vi "数据地址解析.vi"(7 "输入数据":string, 8 "错误输入（无错误）":errorcluster, 9 "地址判断位":bool, 10 "上轮成功输入时间":timestamp, 11 "回传数据队列":refnum<queue>) -> (0 "错误输出":errorcluster, 1 "输出时间":timestamp, 2 "数据状态":string, 3 "回传数据队列":refnum<queue>, 5 "超时标志位":bool)   [LabVIEW 2020]
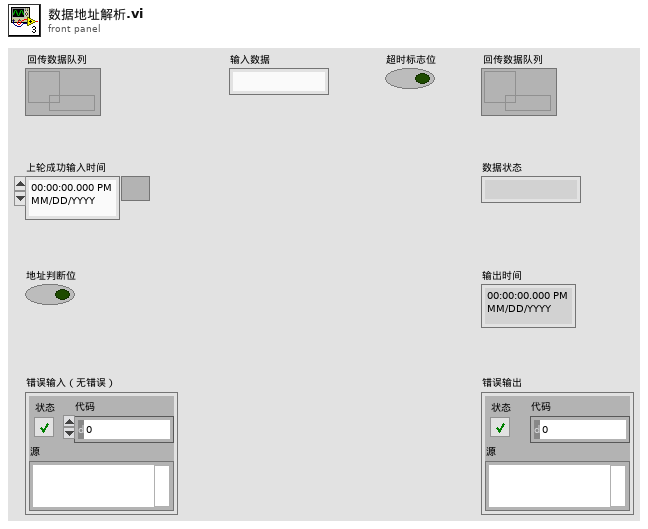
[diagram p1: front panel]
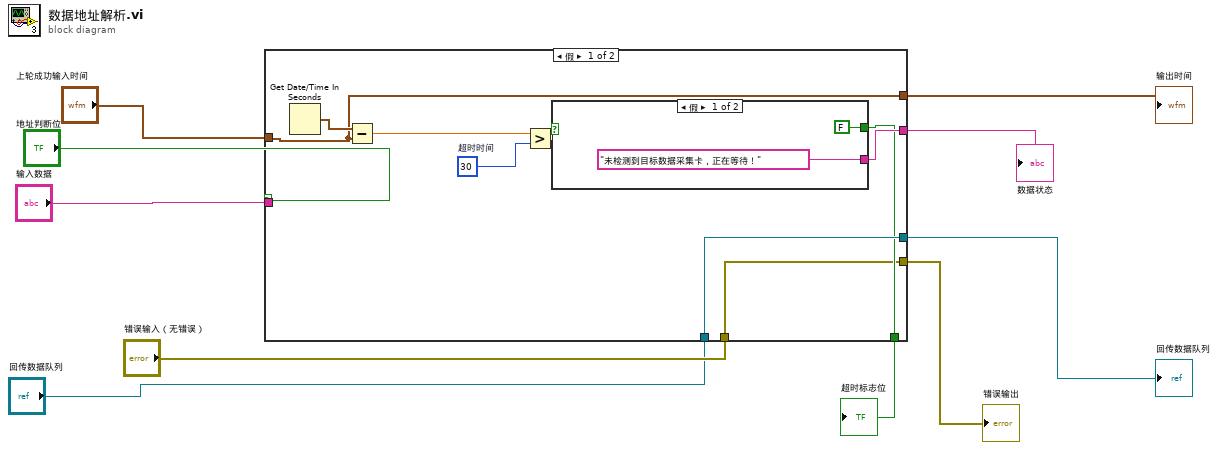
[diagram p0: block diagram]
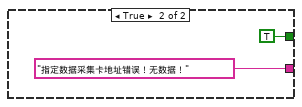
[diagram p2: hidden frame]
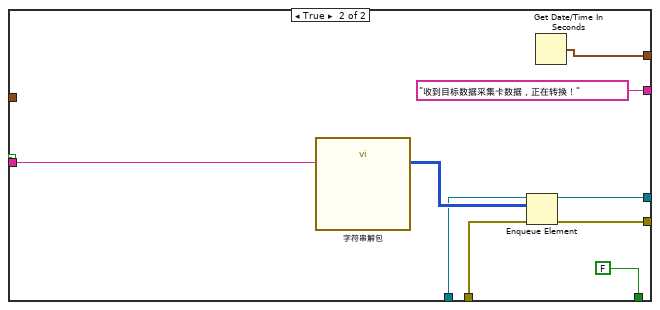
[diagram p3: hidden frame]
diagram:
  n1 = case shown="假" "地址判断位" {
    tunnel: "输入数据" -> [_ w32]
    tunnel: [w15 w30] -> w2
    tunnel: [w12 w29] -> w9
    tunnel: "回传数据队列" -> [w15 w28]
    tunnel: [w14 "收到目标数据采集卡数据，正在转换！"] -> w5
    tunnel: "上轮成功输入时间" -> [w11 _]
    tunnel: [w13 FALSE] -> w7
    tunnel: "错误输入（无错误）" -> [w12 w26]
    tunnel: [w11 w24] -> w10
    frame False {
      w17 = u16 30  # 超时时间
      n2 = Get Date/Time In Seconds() -> (seconds since 1Jan1904=w19:timestamp)
      n3 = Subtract(x=w19, y=w11) -> (x-y=w18:dbl)
      n4 = Greater?(x=w18, y=w17) -> (0:w16:bool)
      n5 = case shown="假" w16 {
        tunnel: ["未检测到目标数据采集卡，正在等待！" "指定数据采集卡地址错误！无数据！"] -> w14
        tunnel: [FALSE TRUE] -> w13
        frame False {
        }
        frame True {
        }
      }
    }
    frame True {
      n6 = call "字符串解包.vi"("data out"=w32) -> ("数组"=w31:i32[][])  [unwired: 10 in]
      n7 = Enqueue Element(queue=w28, element=w31, error in (no error)=w26) -> (queue out=w30:refnum<queue>, error out=w29:errorcluster)  [unwired: 1 in, 1 out]
      n8 = Get Date/Time In Seconds() -> (seconds since 1Jan1904=w24:timestamp)
    }
  }
  "输出时间" <- w10
  "错误输出" <- w9
  "超时标志位" <- w7
  "数据状态" <- w5
  "回传数据队列" <- w2
